vi "Part 1.vi"(11 "Input":string) -> (3 "Output":i64)   [LabVIEW 2021]
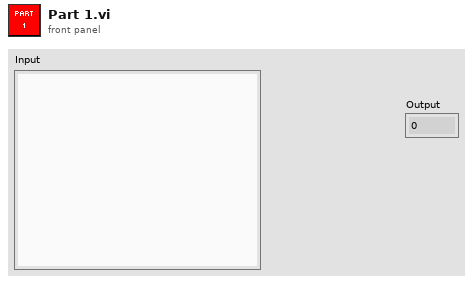
[diagram p1: front panel]
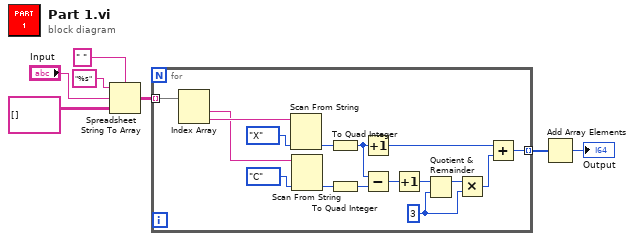
[diagram p0: block diagram]
diagram:
  n1 = Spreadsheet String To Array(delimiter (Tab)=" ", format string="%s", spreadsheet string="Input", array type (2D Dbl)=string[][] []) -> (array=w3:string[][])
  n2 = for {
    tunnel: w3 -> [w23] mode=indexing
    tunnel: [w17] -> w2 mode=indexing
    w14 = i64 3 ("y")
    n3 = Index Array(array=w23) -> (element #1=w20:string, element #2=w22:string)  [unwired: 2 in]
    n4 = Scan From String(input string=w22, default 1=enum16{"X", "Y", "Z"}."X") -> (output 1=w9:enum16{"X", "Y", "Z"})  [unwired: 3 in, 3 out]
    n5 = Scan From String(input string=w20, default 1=enum16{"A", "B", "C"}."C") -> (output 1=w18:enum16{"A", "B", "C"})  [unwired: 3 in, 3 out]
    n6 = To Quad Integer(1:w9) -> (0:w8:i64)
    n7 = To Quad Integer(1:w18) -> (0:w10:i64)
    n8 = Increment(x=w8) -> (x+1=w16:i64)
    n9 = Subtract(x=w8, y=w10) -> (x-y=w11:i64)
    n10 = Increment(x=w11) -> (x+1=w12:i64)
    n11 = Quotient & Remainder(x=w12, y=w14) -> (x-y*floor(x/y)=w13:i64)  [unwired: 1 out]
    n12 = Multiply(x=w13, y=w14) -> (x*y=w15:i64)
    n13 = Add(x=w16, y=w15) -> (x+y=w17:i64)
  }
  n14 = Add Array Elements(numeric array=w2) -> (sum=→"Output":i64)
